vi "flash_RPCV4.vi"() -> ()   [LabVIEW 2017]
panel:
  in  "UDP Update":bool=TRUE
  out "error out 2":errorcluster
  out "Out 2":u8=2 format="%.0x"
  in  "Firmware":u16(ring)=2 items=["TDC"=4, "Middle"=3, "Backend"=2]
  out "Out":u8=1 format="%.0x"
  out "字符串 2":string
  out "concatenated string":string
  in  "Register_Base_Address":u32=512 format="%x"
  in  "start":bool=TRUE
  out "Current IP address":string="10.3.173.20"
  in  "IP address list":string[](array[string])=["10.3.173.20"]
  in  "回读":bool
  out "Current Progress":u32(slide)=6712320 scale=0.0..6712112.0
  out "error out":errorcluster={"status"=TRUE, "code"=1, "source"="TCP Close Connection in flash_RPCV3.vi"}
  out "appended array":bool[](array[boolean])
  out "Process":u32=6712320
  in  "error in (no error)":errorcluster
  in  "Read (TRUE)":bool
  out "byte data":string
  out "Total size (in bytes)":i64=6712112
  in  "bin file path (use dialog)":path=path "G:/rpc/aggregate/WR/firmware/NEM_DEVB/project_1.runs/impl_1/top.bin"
  # "FF80 0001 0000 0209 13"
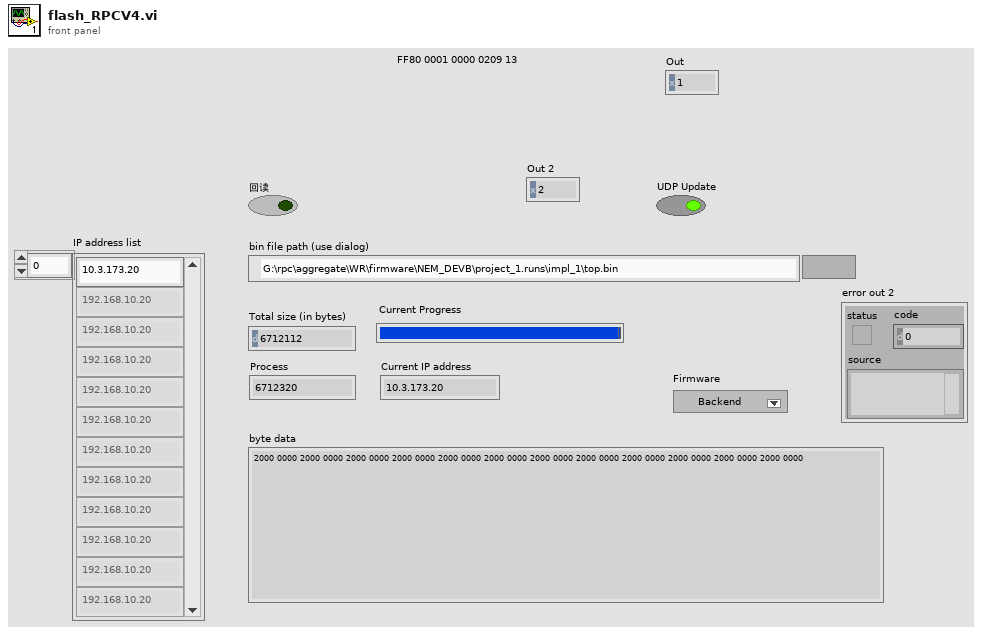
[diagram p1: front panel]
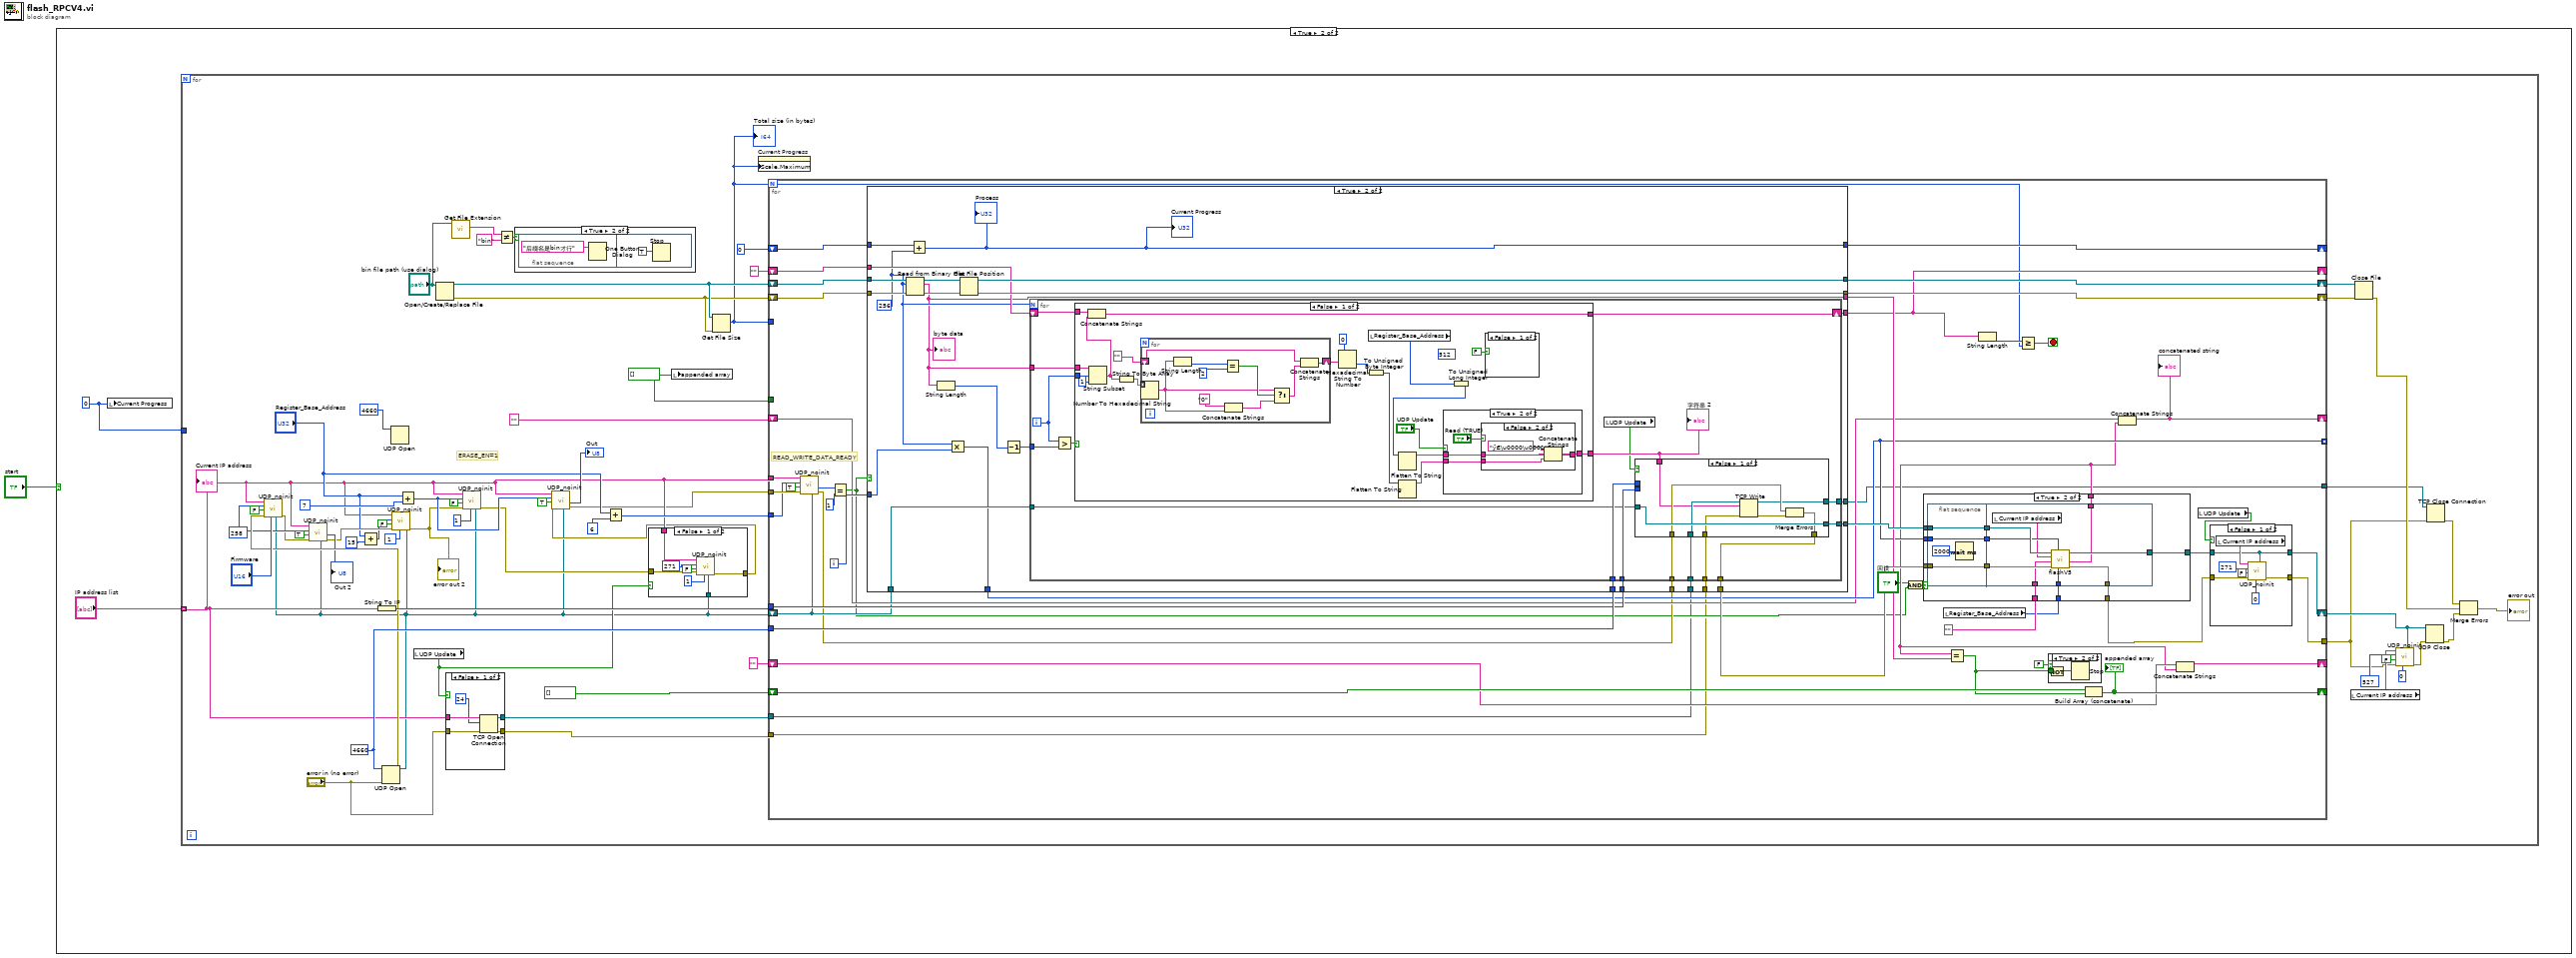
[diagram p0: block diagram]
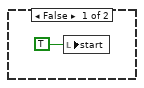
[diagram p2: hidden frame]
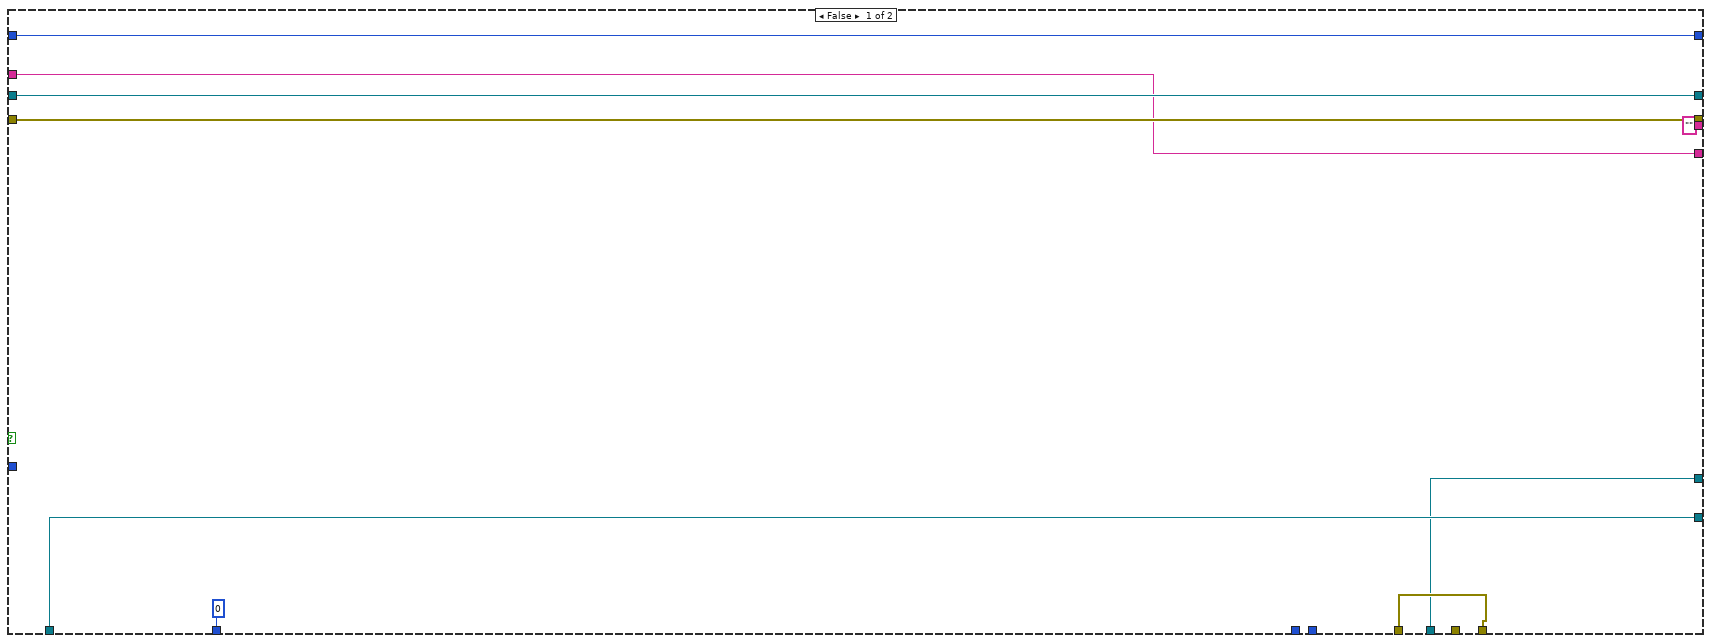
[diagram p7: hidden frame]
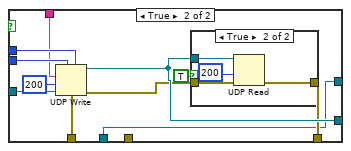
[diagram p8: hidden frame]
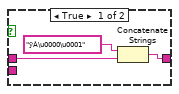
[diagram p11: hidden frame]
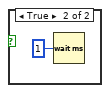
[diagram p12: hidden frame]
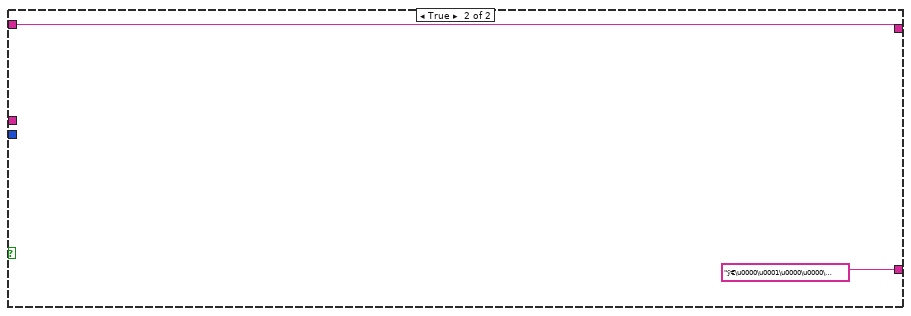
[diagram p13: hidden frame]
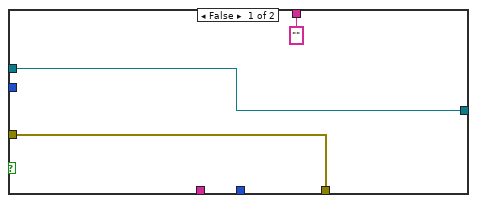
[diagram p14: hidden frame]
diagram:
  n1 = case shown="True" "start" {
    frame False {
      n2 = local write "start"(TRUE ("start")) -> ()
    }
    frame True {
      w3 = u8 0 ("In")
      n3 = local write "Current Progress"(w3) -> ()
      n4 = for {
        tunnel: "IP address list" -> [w13] mode=indexing
        tunnel: w3 -> [_]
        w38 = u32 258 ("Address")
        w51 = bool[] [] ("appended array")
        w61 = u16 4660 ("UDP port")
        # "ERASE_EN=1"
        n5 = Add(x="Register_Base_Address", y=u32 15 ("Address")) -> (x+y=w26:u32)
        n6 = String To IP(1:w13) -> (0:w60:u32)
        n7 = UDP Open(8:"error in (no error)", 11:w61) -> (port=w5:refnum<k16>, 0:w39:errorcluster)  [unwired: 3 in, 1 out]
        n8 = call "UDP_noinit.vi"("connection ID"=w5, "In"="Firmware", "error in (no error)"=w39, "Read (TRUE)"=FALSE, "Address"=w38, "IP address"=w13) -> ("error out"=w35:errorcluster)  [unwired: 2 in, 2 out]
        n9 = call "UDP_noinit.vi"("connection ID"=w5, "error in (no error)"=w35, "Read (TRUE)"=TRUE, "Address"=w38, "IP address"=w13) -> ("error out"=w28:errorcluster, "Out"=→"Out 2":u8)  [unwired: 3 in, 1 out]
        n10 = UDP Open(11:u16 4660 ("UDP port")) -> ()  [unwired: 4 in, 3 out]
        n11 = call "UDP_noinit.vi"("connection ID"=w5, "In"=u32 1 ("Address"), "error in (no error)"=w28, "Read (TRUE)"=FALSE, "Address"=w26, "IP address"=w13) -> ("error out"=w27:errorcluster)  [unwired: 2 in, 2 out]
        "error out 2" <- w27
        n12 = Add(x="Register_Base_Address", y=u32 7 ("Address")) -> (x+y=w46:u32)
        n13 = local read "UDP Update"() -> (w14:bool)
        n14 = Open/Create/Replace File(file path (use dialog)="bin file path (use dialog)") -> (refnum out=w65:refnum<file>, error out=w64:errorcluster)  [unwired: 5 in, 1 out]
        n15 = case shown="False" w14 {
          tunnel: w13 -> [w80 _]
          tunnel: "error in (no error)" -> [w78 w81]
          tunnel: [w77 _] -> w19
          tunnel: [w76 w81] -> w18
          frame False {
            n16 = TCP Open Connection(address=w80, remote port or service name=u16 24 ("UDP port"), error in (no error)=w78) -> (connection ID=w77:refnum<k5>, error out=w76:errorcluster)  [unwired: 2 in]
          }
          frame True {
          }
        }
        n17 = call <vilib>:"Get File Extension.vi"("file"="bin file path (use dialog)") -> ("lowercase file extension"=w11:string)  [unwired: 6 in, 4 out]
        n18 = call "UDP_noinit.vi"("connection ID"=w5, "In"=u8 1, "error in (no error)"=w27, "Read (TRUE)"=FALSE, "Address"=w46, "IP address"=w13) -> ("error out"=w8:errorcluster)  [unwired: 2 in, 2 out]
        n19 = Not Equal?(x=w11, y="bin") -> (x != y?=w9:bool)
        n20 = case shown="True" w9 {
          frame False {
          }
          frame True {
            n21 = flat-sequence {
              frame #0 {
                n22 = One Button Dialog(message="后缀名是bin才行") -> ()  [unwired: 1 in, 1 out]
              }
              frame #1 {
                n23 = Stop(stop? (T)=TRUE) -> ()
              }
            }
          }
        }
        n24 = Add(x="Register_Base_Address", y=u32 6 ("Address")) -> (x+y=w44:u32)
        n25 = case shown="False" w14 {
          tunnel: w8 -> [w74 w75]
          tunnel: w13 -> [w73 _]
          tunnel: [w70 w75] -> w7
          tunnel: w5 -> [w68 _]
          frame False {
            n26 = call "UDP_noinit.vi"("connection ID"=w68, "In"=u8 1, "error in (no error)"=w74, "Read (TRUE)"=FALSE, "Address"=u32 271, "IP address"=w73) -> ("error out"=w70:errorcluster)  [unwired: 2 in, 2 out]
          }
          frame True {
          }
        }
        n27 = call "UDP_noinit.vi"("connection ID"=w5, "error in (no error)"=w7, "Read (TRUE)"=TRUE, "Address"=w46, "IP address"=w13) -> ("error out"=w6:errorcluster, "Out"=→"Out":u8)  [unwired: 3 in, 1 out]
        n28 = local write "appended array"(w51) -> ()
        n29 = Get File Size(file=w65, error in=w64) -> (size (in bytes)=w52:i64)  [unwired: 2 out]
        "Total size (in bytes)" <- w52
        n30 = property on="Current Progress" class="Slide (strict)"("Scale.Maximum"=w52) -> ()  [unwired: 2 in, 2 out]
        n31 = for {
          N: w52 -> [w109]
          tunnel: w52 -> [_]
          shift-right: [w127] -> w63
          shift-left: w64 -> [w128]
          shift-right: [w126] -> w62
          shift-left: w65 -> [w129]
          shift-right: [w111] -> _
          shift-left: "" -> [w125]
          tunnel: w61 -> [w122]
          tunnel: [w83] -> w16
          tunnel: w60 -> [w121]
          shift-right: [w82] -> w30
          shift-left: w5 -> [w99]
          shift-right: [w123] -> _
          shift-left: u32 0 ("length (rest)") -> [w124]
          shift-right: [w116] -> _
          shift-left: bool[] [] -> [w114]
          tunnel: [w112] -> _ mode=indexing
          shift-right: [w107] -> _
          shift-left: "" -> [w106]
          tunnel: w13 -> [w104]
          tunnel: w6 -> [w98]
          shift-right: [w96] -> _
          shift-left: "" -> [w95]
          tunnel: w51 -> [_]
          tunnel: w44 -> [w91]
          tunnel: w19 -> [w89]
          tunnel: w18 -> [w88]
          tunnel: [w87] -> w17
          i -> [w117]
          stop <- w108 stop-if-true
          # "READ_WRITE_DATA_READY"
          n32 = call "UDP_noinit.vi"("connection ID"=w99, "error in (no error)"=w98, "Read (TRUE)"=TRUE, "Address"=w91, "IP address"=w104) -> ("error out"=w97:errorcluster, "Out"=w102:u8)  [unwired: 3 in, 1 out]
          n33 = Equal?(x=w102, y=u8 1) -> (x = y?=w93:bool)
          n34 = case shown="True" w93 {
            tunnel: w129 -> [w144 w172]
            tunnel: w128 -> [w145 w171]
            tunnel: [w145 w168] -> w127
            tunnel: [w144 w167] -> w126
            tunnel: w125 -> [w142 w166]
            tunnel: w124 -> [w143 w165]
            tunnel: [w143 w151] -> w123
            tunnel: w122 -> [_ w164]
            tunnel: w121 -> [_ w163]
            tunnel: w97 -> [w146 w162]
            tunnel: w99 -> [w147 w161]
            tunnel: [w147 w158] -> w120
            tunnel: [w146 w157] -> w119
            tunnel: w117 -> [_ w156]
            tunnel: ["" w154] -> w115
            tunnel: [0 w153] -> w112
            tunnel: [w142 w152] -> w111
            tunnel: w89 -> [w139 w150]
            tunnel: w88 -> [_ w149]
            tunnel: [w139 w148] -> w87
            frame False {
            }
            frame True {
              w155 = 256 ("count (1)")
              n35 = Read from Binary File(8:w171, 10:w155, 11:w172) -> (0:w169:errorcluster, 2:w154:string, 3:w170:refnum<file>)  [unwired: 3 in, 1 out]
              "byte data" <- w154
              n36 = Add(x=w165, y=w155) -> (x+y=w151:u32)
              "Process" <- w151
              "Current Progress" <- w151
              n37 = String Length(string=w154) -> (length=w160:i32)
              n38 = Multiply(x=w155, y=w156) -> (x*y=w153:i32)
              n39 = Get File Position(4:w169, 7:w170) -> (0:w168:errorcluster, 3:w167:refnum<file>)  [unwired: 1 out]
              n40 = Decrement(x=w160) -> (x-1=w159:i32)
              n41 = for {
                N: w155 -> [_]
                tunnel: w154 -> [w189]
                shift-right: [w187] -> w152
                shift-left: w166 -> [w188]
                tunnel: w164 -> [w186]
                tunnel: w163 -> [w185]
                tunnel: w162 -> [w184]
                tunnel: w161 -> [w179]
                tunnel: [w177] -> w157
                tunnel: [w178] -> w158
                tunnel: w159 -> [w182]
                tunnel: w150 -> [w175]
                tunnel: w149 -> [w174]
                tunnel: [w173] -> w148
                i -> [w181]
                n42 = Greater?(x=w181, y=w182) -> (0:w183:bool)
                n43 = case shown="False" w183 {
                  tunnel: w189 -> [w225 _]
                  tunnel: w188 -> [w223 w256]
                  tunnel: [w222 w256] -> w187
                  tunnel: w181 -> [w217 _]
                  tunnel: [w216 "ÿ€\u0000\u0001\u0000\u0000\u0000@\u0000" ("字符串 2")] -> w180
                  frame False {
                    (unwired) u32 512 ("Address")
                    n44 = String Subset(string=w225, offset (0)=w217, length (rest)=1 ("length (rest)")) -> (substring=w221:string)
                    n45 = Concatenate Strings(w223, w221) -> (w222:string)
                    n46 = String To Byte Array(string=w221) -> (unsigned byte array=w231:u8[])
                    n47 = for {
                      shift-right: [w254] -> w230
                      shift-left: "" ("format string") -> [w251]
                      tunnel: w231 -> [w255] mode=indexing
                      n48 = Number To Hexadecimal String(2:w255) -> (0:w247:string)  [unwired: 1 in]
                      n49 = String Length(string=w247) -> (length=w253:i32)
                      n50 = Equal?(x=w253, y=2) -> (x = y?=w250:bool)
                      n51 = Concatenate Strings("0" ("format string"), w247) -> (w249:string)
                      n52 = Select(t=w247, s=w250, f=w249) -> (s? t:f=w246:string)
                      n53 = Concatenate Strings(w251, w246) -> (w254:string)
                    }
                    n54 = Hexadecimal String To Number(string=w230, default (0uL)=u64 0 ("default (0 U32)")) -> (number=w228:u64)  [unwired: 1 in, 1 out]
                    n55 = To Unsigned Byte Integer(number=w228) -> (unsigned 8bit integer=w227:u8)
                    n56 = local read "Register_Base_Address"() -> (w215:u32)
                    n57 = Flatten To String(anything=w227) -> (data string=w218:string)  [unwired: 3 in, 2 out]
                    n58 = To Unsigned Long Integer(number=w215) -> (unsigned 32bit integer=w226:u32)
                    n59 = Flatten To String(anything=w226) -> (data string=w219:string)  [unwired: 3 in, 2 out]
                    n60 = case shown="True" "UDP Update" {
                      tunnel: w219 -> [_ w237]
                      tunnel: w218 -> [w233 w236]
                      tunnel: [w233 w234] -> w216
                      frame False {
                      }
                      frame True {
                        n61 = case shown="False" "Read (TRUE)" {
                          tunnel: [w239 w243] -> w234
                          tunnel: w237 -> [w238 w242]
                          tunnel: w236 -> [_ w241]
                          frame True {
                            n62 = Concatenate Strings("ÿÀ\u0000\u0001" ("initial string"), w238) -> (w239:string)
                          }
                          frame False {
                            n63 = Concatenate Strings("ÿ€\u0000\u0001" ("initial string"), w242, w241) -> (w243:string)
                          }
                        }
                      }
                    }
                    n64 = case shown="False" FALSE {
                      frame False {
                      }
                      frame True {
                        n65 = Wait (ms)(milliseconds to wait=u32 1) -> ()  [unwired: 1 out]
                      }
                    }
                  }
                  frame True {
                  }
                }
                "字符串 2" <- w180
                n66 = local read "UDP Update"() -> (w176:bool)
                n67 = case shown="False" w176 {
                  tunnel: w186 -> [_ w208]
                  tunnel: w185 -> [_ w207]
                  tunnel: w184 -> [w194 w206]
                  tunnel: w180 -> [w191 w204]
                  tunnel: w179 -> [w197 w203]
                  tunnel: [w197 w202] -> w178
                  tunnel: [w192 w199] -> w177
                  tunnel: w175 -> [w196 w198]
                  tunnel: w174 -> [w195 _]
                  tunnel: [w190 w198] -> w173
                  frame False {
                    n68 = TCP Write(connection ID=w196, data in=w191, error in (no error)=w195) -> (connection ID out=w190:refnum<k5>, error out=w193:errorcluster)  [unwired: 1 in, 1 out]
                    n69 = Merge Errors(w194, w193) -> (w192:errorcluster)
                  }
                  frame True {
                    n70 = UDP Write(address=w207, port or service name=w208, connection ID=w203, data in=w204, 8:w206, 9:200 ("timeout ms (25000)")) -> (error out=w200:errorcluster, 3:w202:refnum<k16>)
                    n71 = case shown="True" TRUE {
                      tunnel: w202 -> [_ w213]
                      tunnel: w200 -> [w209 w212]
                      tunnel: [w209 w211] -> w199
                      frame False {
                      }
                      frame True {
                        n72 = UDP Read(connection ID=w213, timeout ms (25000)=200, 8:w212) -> (error out=w211:errorcluster)  [unwired: 5 out]
                      }
                    }
                  }
                }
              }
            }
          }
          n73 = And(x="回读", y=w93) -> (x .and. y?=w100:bool)
          n74 = local read "Register_Base_Address"() -> (w90:u32)
          n75 = case shown="True" w100 {
            tunnel: w120 -> [w260 w268]
            tunnel: [w260 w267] -> w86
            tunnel: w119 -> [w259 w266]
            tunnel: [w259 w265] -> w84
            tunnel: "" ("empty") -> [_ w264]
            tunnel: w112 -> [_ w263]
            tunnel: ["" ("String") w262] -> w94
            tunnel: w90 -> [_ w261]
            frame False {
            }
            frame True {
              n76 = flat-sequence {
                tunnel: w263 -> [w273]
                tunnel: w266 -> [w274]
                tunnel: w268 -> [w275]
                tunnel: [w275] -> w271
                tunnel: [w274] -> w270
                tunnel: [w273] -> w269
                tunnel: [w281] -> w265
                tunnel: w264 -> [w280]
                tunnel: [w279] -> w262
                tunnel: w271 -> [w284]
                tunnel: w270 -> [w282]
                tunnel: w269 -> [w278]
                tunnel: [w283] -> w267
                tunnel: w261 -> [w276]
                frame #0 {
                  n77 = Wait (ms)(milliseconds to wait=u32 2000) -> ()  [unwired: 1 out]
                }
                frame #1 {
                  n78 = local read "Current IP address"() -> (w277:string)
                  n79 = call "flashV5.vi"("Register_Base_Address"=w276, "flash_base_address"=w278, "error in (no error)"=w282, "empty"=w280, "address"=w277, "connection ID"=w284) -> ("error out"=w281:errorcluster, "String"=w279:string, "connection ID 2"=w283:refnum<k16>)  [unwired: 2 in, 1 out]
                }
              }
            }
          }
          n80 = Equal?(x=w94, y=w115) -> (x = y?=w113:bool)
          n81 = String Length(string=w111) -> (length=w110:i32)
          n82 = Greater Or Equal?(x=w110, y=w109) -> (x >= y?=w108:bool)
          n83 = case shown="True" FALSE {
            tunnel: w113 -> [_ w285]
            frame False {
            }
            frame True {
              n84 = Not(x=w285) -> (.not. x?=w286:bool)
              n85 = Stop(stop? (T)=w286) -> ()
            }
          }
          n86 = Build Array (concatenate)(w114, w113) -> (w116:bool[])
          "appended array" <- w116
          n87 = Concatenate Strings(w106, w94) -> (w107:string)
          "concatenated string" <- w107
          n88 = Concatenate Strings(w95, w94) -> (w96:string)
          n89 = local read "UDP Update"() -> (w85:bool)
          n90 = case shown="False" w85 {
            tunnel: w86 -> [w130 w137]
            tunnel: w84 -> [w136 w138]
            tunnel: [w135 w138] -> w83
            tunnel: [w130 w137] -> w82
            frame False {
              n91 = local read "Current IP address"() -> (w134:string)
              n92 = call "UDP_noinit.vi"("connection ID"=w130, "In"=u8 0, "error in (no error)"=w136, "Read (TRUE)"=FALSE, "Address"=u32 271, "IP address"=w134) -> ("error out"=w135:errorcluster)  [unwired: 2 in, 2 out]
            }
            frame True {
            }
          }
        }
        n93 = local read "Current IP address"() -> (w32:string)
        n94 = Close File(refnum=w62, error in=w63) -> (error out=w50:errorcluster)  [unwired: 1 out]
        n95 = call "UDP_noinit.vi"("connection ID"=w30, "In"=u8 0, "error in (no error)"=w16, "Read (TRUE)"=FALSE, "Address"=u32 527, "IP address"=w32) -> ("error out"=w31:errorcluster)  [unwired: 2 in, 2 out]
        n96 = UDP Close(connection ID=w30, 8:w31) -> (error out=w49:errorcluster)  [unwired: 1 out]
        n97 = TCP Close Connection(connection ID=w17, error in (no error)=w16) -> (error out=w15:errorcluster)  [unwired: 1 in, 1 out]
        n98 = Merge Errors(w15, w50, w49) -> (→"error out":errorcluster)
        "Current IP address" <- w13
      }
    }
  }
